vi "Stop Core.vi"(10 "final error code":i32, 11 "SLZ-KA1 in":refnum<class "SLZ-KA1.lvclass">) -> (3 "SLZ-KA1 out":refnum<class "SLZ-KA1.lvclass">)   [LabVIEW 2015, in "SLZ-KA1 Actor.lvlib" / "SLZ-KA1.lvclass"]
doc: "(<B>Filename</B>: Actor Framework.lvlib:Actor.lvclass:Stop Core.vi)\n\nDefines what the actor does before it stops. Use the <B>final error code</B> input to determine whether the actor shut down in response to an error.\n\nBy default, this method does nothing. A descendant class may override it to define behavior, such as shutting down any processes the actor initiated in its override of the Actor Core method."
uses:
  SLZ-KA1.lvclass
  SLZ-KA1.lvclass/SLZ-KA1.ctl
  <vilib>/ActorFramework/Actor/Actor.lvclass
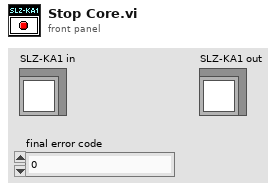
[diagram p1: front panel]
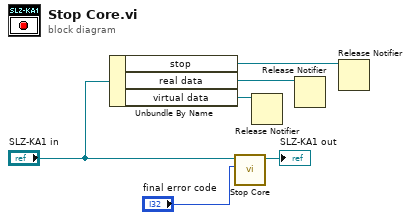
[diagram p0: block diagram]
diagram:
  n1 = Unbundle By Name("SLZ-KA1 in") -> ("stop"=w2:refnum<notifier>, "real data"=w3:refnum<notifier>, "virtual data"=w1:refnum<notifier>)
  n2 = call-parent "Stop Core.vi"("final error code"="final error code", "Actor in"="SLZ-KA1 in") -> ("Actor out"=→"SLZ-KA1 out":refnum<class "SLZ-KA1.lvclass">)  [unwired: 9 in]
  n3 = Release Notifier(notifier=w1) -> ()  [unwired: 2 in, 3 out]
  n4 = Release Notifier(notifier=w3) -> ()  [unwired: 2 in, 3 out]
  n5 = Release Notifier(notifier=w2) -> ()  [unwired: 2 in, 3 out]
